vi "Delete CHM Files.vi"(8 "error in (no error)":errorcluster, 11 "Path":path) -> (0 "error out":errorcluster)   [LabVIEW 2022 SP3]
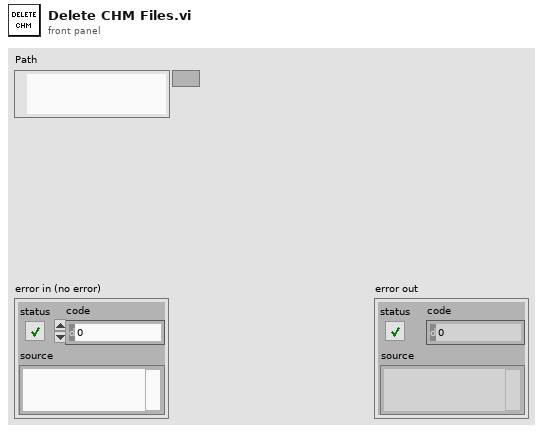
[diagram p1: front panel]
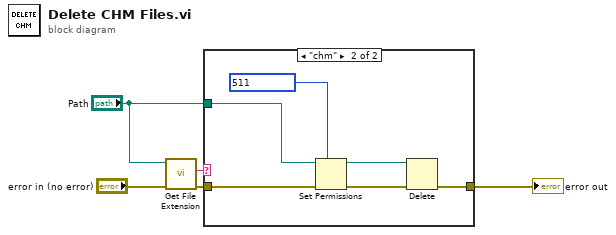
[diagram p0: block diagram]
diagram:
  n1 = call <vilib>:"Get File Extension.vi"("error in (no error)"="error in (no error)", "file"="Path") -> ("error out"=w3:errorcluster, "lowercase file extension"=w4:string)  [unwired: 5 in, 3 out]
  n2 = case shown="\"chm\"" w4 {
    tunnel: w3 -> [w6 w11]
    tunnel: [w6 w12] -> w2
    tunnel: "Path" -> [_ w9]
    frame "", Default {
    }
    frame "chm" {
      n3 = Set Permissions(7:i16 511 ("permissions"), 8:w11, 11:w9) -> (0:w10:errorcluster, 3:w8:path)  [unwired: 2 in]
      n4 = Delete(path (use dialog)=w8, error in=w10) -> (error out=w12:errorcluster)  [unwired: 3 in, 2 out]
    }
  }
  "error out" <- w2
